vi "Convert Analog Measurement to Analog PWM.vi"(1 "Analog PWM Measurement":T1) -> (0 "Analog PWM Values":dbl[](array[numeric]))   [LabVIEW 2018, in "FPGA Addon Engine.lvlib"]
uses:
  FPGA Addon Engine.lvlib
  Submodules/Source/Types/PWM.Measure.Analog.Measurement.ctl
  Submodules/Source/Speciality FPGA IO.lvlib
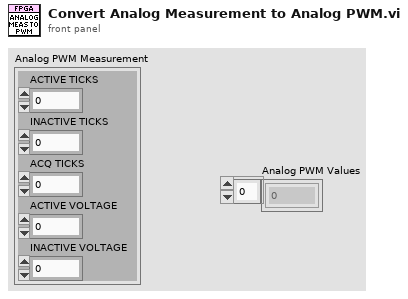
[diagram p1: front panel]
types:
  T1 = typedef "Speciality FPGA IO.lvlib/PWM.Measure.Analog.Measurement.ctl" = cluster{"ACTIVE TICKS":u32, "INACTIVE TICKS":u32, "ACQ TICKS":u32, "ACTIVE VOLTAGE":fxp<+/-,32,8>, "INACTIVE VOLTAGE":fxp<+/-,32,8>}
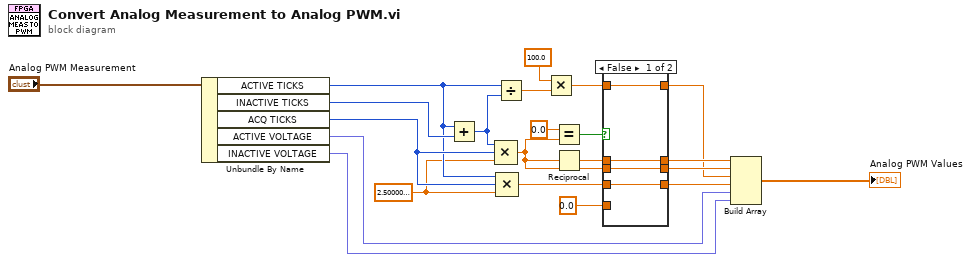
[diagram p0: block diagram]
diagram:
  w6 = 2.5000000292152436e-08 ("y")
  n1 = Unbundle By Name("Analog PWM Measurement") -> ("ACTIVE TICKS"=w15:u32, "INACTIVE TICKS"=w16:u32, "ACQ TICKS"=w17:u32, "ACTIVE VOLTAGE"=w18:fxp<+/-,32,8>, "INACTIVE VOLTAGE"=w19:fxp<+/-,32,8>)
  n2 = Add(x=w15, y=w16) -> (x+y=w4:u32)
  n3 = Compound Arithmetic op=MULTIPLY(w4, w17, w6) -> (w3:dbl)
  n4 = Divide(x=w15, y=w4) -> (x/y=w10:dbl)
  n5 = Compound Arithmetic op=MULTIPLY(w15, w17, w6) -> (w5:dbl)
  n6 = Multiply(x=100.0, y=w10) -> (x*y=w11:dbl)
  n7 = Equal?(x=0.0, y=w3) -> (x = y?=w7:bool)
  n8 = Reciprocal(x=w3) -> (1/x=w2:dbl)
  n9 = case shown="False" w7 {
    tunnel: [w23 w27] -> w20
    tunnel: [w24 w27] -> w14
    tunnel: [w26 w27] -> w21
    tunnel: w3 -> [w26 _]
    tunnel: [w25 w27] -> w12
    tunnel: w5 -> [w25 _]
    tunnel: w11 -> [w24 _]
    tunnel: w2 -> [w23 _]
    tunnel: 0.0 ("x") -> [_ w27]
    frame False {
    }
    frame True {
    }
  }
  n10 = Build Array(w20, w21, w14, w12, w18, w19) -> (→"Analog PWM Values":dbl[])
